vi "Run Me.vi"() -> ()   [LabVIEW 2020]
uses:
  Interfaces/DMM HAL/rwr_Read Measurement Reply.ctl
  Workers/Fluke DMM/Fluke DMM.lvclass
  Interfaces/DMM HAL/DMM HAL.lvclass
  Workers/Keithley DMM/Keithley DMM.lvclass
panel:
  out "Running":bool
  out "Running":bool
  in  "Stop Keithley DMM":bool
  out "Reply Data Keithley":T1
  out "Reply Data Fluke":T1
  in  "Stop Fluke DMM":bool
  # "FLUKE DMM"
  # "KEITHLEY DMM"
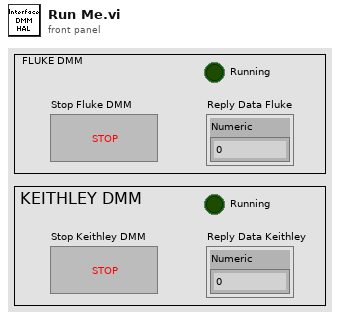
[diagram p1: front panel]
types:
  T1 = typedef "DMM HAL.lvclass/rwr_Read Measurement Reply.ctl" = cluster{"Numeric":dbl}
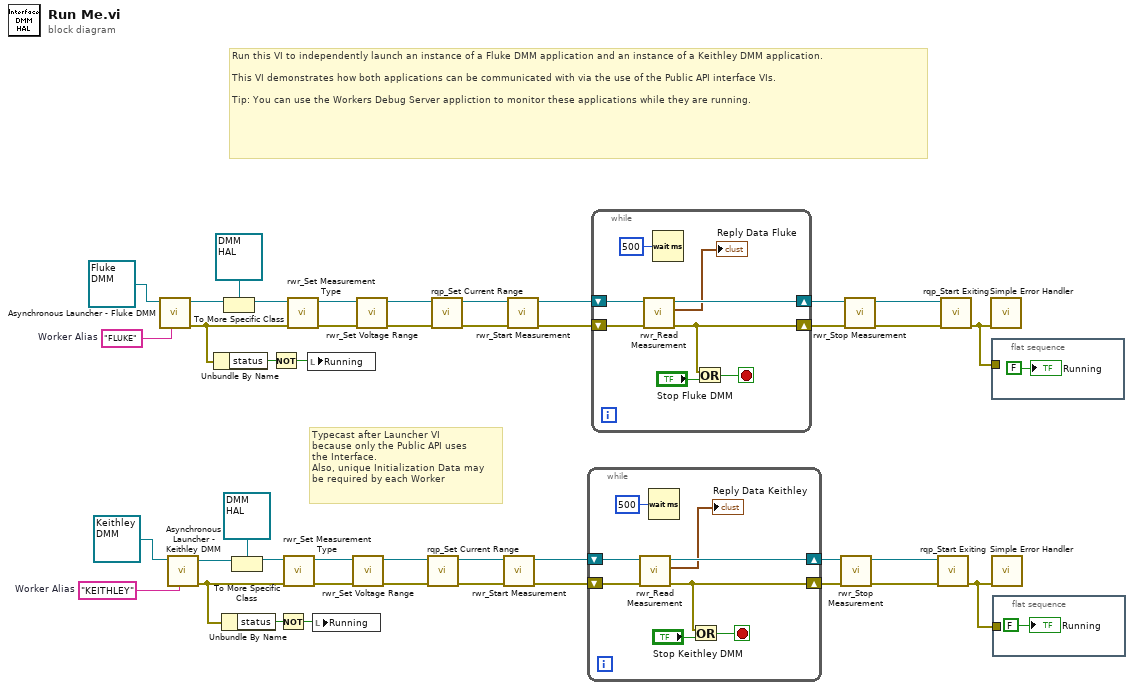
[diagram p0: block diagram]
diagram:
  w16 = "KEITHLEY"  # Worker Alias
  w35 = "FLUKE"  # Worker Alias
  # "Run this VI to independently launch an instance of a Fluke DMM application and an instance of a Keithley DMM application.\n\nThis VI demonstrates how both applications can be communicated with via the use of the Public API interface VIs.\n\nTip: You can use the Workers Debug Server appliction to monitor these applications while they are running."
  # "Typecast after Launcher VI\nbecause only the Public API uses \nthe Interface.\nAlso, unique Initialization Data may \nbe required by each Worker"
  n1 = call "Asynchronous Launcher - Fluke DMM.vi"("Worker Alias"=w35, "Fluke DMM in"=refnum<class "Fluke DMM.lvclass"> refnum ("Fluke DMM")) -> ("error out"=w5:errorcluster, "Fluke DMM out"=w36:refnum<class "Fluke DMM.lvclass">)  [unwired: 8 in]
  n2 = call "Asynchronous Launcher - Keithley DMM.vi"("Worker Alias"=w16, "Fluke DMM in"=refnum<class "Keithley DMM.lvclass"> refnum ("Fluke DMM")) -> ("error out"=w8:errorcluster, "Fluke DMM out"=w10:refnum<class "Keithley DMM.lvclass">)  [unwired: 8 in]
  n3 = Unbundle By Name(w5) -> ("status"=w6:bool)
  n4 = Unbundle By Name(w8) -> ("status"=w7:bool)
  n5 = To More Specific Class(target class=refnum<class "DMM HAL.lvclass"> refnum ("Interface 1.lvclass"), reference=w36) -> (specific class reference=w14:refnum<class "DMM HAL.lvclass">)  [unwired: 1 in, 1 out]
  n6 = To More Specific Class(target class=refnum<class "DMM HAL.lvclass"> refnum ("Interface 1.lvclass"), reference=w10) -> (specific class reference=w11:refnum<class "DMM HAL.lvclass">)  [unwired: 1 in, 1 out]
  n7 = Not(x=w6) -> (.not. x?=w4:bool)
  n8 = Not(x=w7) -> (.not. x?=w3:bool)
  n9 = call-dynamic "rwr_Set Measurement Type.vi"("error in"=w8, "DMM HAL in"=w11) -> ("error out"=w24:errorcluster, "dup DMM HAL out"=w23:refnum<class "DMM HAL.lvclass">)  [unwired: 7 in, 1 out]
  n10 = call-dynamic "rwr_Set Measurement Type.vi"("error in"=w5, "DMM HAL in"=w14) -> ("error out"=w33:errorcluster, "dup DMM HAL out"=w34:refnum<class "DMM HAL.lvclass">)  [unwired: 7 in, 1 out]
  n11 = local write "Running"(w4) -> ()
  n12 = local write "Running"(w3) -> ()
  n13 = call-dynamic "rwr_Set Voltage Range.vi"("error in"=w24, "DMM HAL in"=w23) -> ("error out"=w25:errorcluster, "dup DMM HAL out"=w27:refnum<class "DMM HAL.lvclass">)  [unwired: 7 in, 1 out]
  n14 = call-dynamic "rwr_Set Voltage Range.vi"("error in"=w33, "DMM HAL in"=w34) -> ("error out"=w32:errorcluster, "dup DMM HAL out"=w30:refnum<class "DMM HAL.lvclass">)  [unwired: 7 in, 1 out]
  n15 = call-dynamic "rqp_Set Current Range.vi"("error in"=w25, "DMM HAL in"=w27) -> ("error out"=w26:errorcluster, "dup DMM HAL out"=w28:refnum<class "DMM HAL.lvclass">)  [unwired: 8 in]
  n16 = call-dynamic "rqp_Set Current Range.vi"("error in"=w32, "DMM HAL in"=w30) -> ("error out"=w31:errorcluster, "dup DMM HAL out"=w29:refnum<class "DMM HAL.lvclass">)  [unwired: 8 in]
  n17 = call-dynamic "rwr_Start Measurement.vi"("error in"=w26, "DMM HAL in"=w28) -> ("error out"=w18:errorcluster, "dup DMM HAL out"=w17:refnum<class "DMM HAL.lvclass">)  [unwired: 7 in, 1 out]
  n18 = call-dynamic "rwr_Start Measurement.vi"("error in"=w31, "DMM HAL in"=w29) -> ("error out"=w41:errorcluster, "dup DMM HAL out"=w42:refnum<class "DMM HAL.lvclass">)  [unwired: 7 in, 1 out]
  n19 = while {
    shift-right: [w48] -> w19
    shift-left: w17 -> [w50]
    shift-right: [w46] -> w20
    shift-left: w18 -> [w49]
    stop <- w45 stop-if-true
    n20 = call-dynamic "rwr_Read Measurement.vi"("error in"=w49, "DMM HAL in"=w50) -> ("error out"=w46:errorcluster, "Reply Data out"=→"Reply Data Keithley":T1, "dup DMM HAL out"=w48:refnum<class "DMM HAL.lvclass">)  [unwired: 7 in]
    n21 = Wait (ms)(milliseconds to wait=u32 500) -> ()  [unwired: 1 out]
    n22 = Or(x=w46, y="Stop Keithley DMM") -> (x .or. y?=w45:bool)
  }
  n23 = while {
    shift-right: [w56] -> w40
    shift-left: w42 -> [w58]
    shift-right: [w54] -> w39
    shift-left: w41 -> [w57]
    stop <- w53 stop-if-true
    n24 = call-dynamic "rwr_Read Measurement.vi"("error in"=w57, "DMM HAL in"=w58) -> ("error out"=w54:errorcluster, "Reply Data out"=→"Reply Data Fluke":T1, "dup DMM HAL out"=w56:refnum<class "DMM HAL.lvclass">)  [unwired: 7 in]
    n25 = Wait (ms)(milliseconds to wait=u32 500) -> ()  [unwired: 1 out]
    n26 = Or(x=w54, y="Stop Fluke DMM") -> (x .or. y?=w53:bool)
  }
  n27 = call-dynamic "rwr_Stop Measurement.vi"("error in"=w20, "DMM HAL in"=w19) -> ("error out"=w22:errorcluster, "dup DMM HAL out"=w21:refnum<class "DMM HAL.lvclass">)  [unwired: 7 in, 1 out]
  n28 = call-dynamic "rwr_Stop Measurement.vi"("error in"=w39, "DMM HAL in"=w40) -> ("error out"=w37:errorcluster, "dup DMM HAL out"=w38:refnum<class "DMM HAL.lvclass">)  [unwired: 7 in, 1 out]
  n29 = call-dynamic "rqp_Start Exiting.vi"("error in"=w22, "DMM HAL in"=w21) -> ("error out"=w1:errorcluster)  [unwired: 8 in, 1 out]
  n30 = call-dynamic "rqp_Start Exiting.vi"("error in"=w37, "DMM HAL in"=w38) -> ("error out"=w2:errorcluster)  [unwired: 8 in, 1 out]
  n31 = call <vilib>:"Simple Error Handler.vi"("error in (no error)"=w2) -> ()  [unwired: 4 in, 5 out]
  n32 = flat-sequence {
    tunnel: w2 -> [_]
    frame #0 {
      "Running" <- FALSE ("Running")
    }
  }
  n33 = call <vilib>:"Simple Error Handler.vi"("error in (no error)"=w1) -> ()  [unwired: 4 in, 5 out]
  n34 = flat-sequence {
    tunnel: w1 -> [_]
    frame #0 {
      "Running" <- FALSE ("Running")
    }
  }
